vi "Init Condition.vi"(5 "Sequencing":refnum<class "MessageQ.lvclass">, 6 "Variables":refnum<class "Variables.lvclass">, 7 "VolatusAPI":refnum<class "VolatusAPI.lvclass">, 8 "error in (no error)":refnum<class "MultiErrors.lvclass">, 10 "Condition Config":refnum<class "Condition Config.lvclass">, 11 "OutOfRange Condition in":refnum<class "OutOfRange Condition.lvclass">) -> (0 "error out":refnum<class "MultiErrors.lvclass">, 3 "OutOfRange Condition out":refnum<class "OutOfRange Condition.lvclass">)   [LabVIEW 2020, in "VolatusSeq.lvlib" / "OutOfRange Condition.lvclass"]
uses:
  OutOfRange Condition.lvclass
  VolatusErrorUtilities/MultiErrors/MultiErrors.lvclass
  Volatus/VolatusAPI/VolatusAPI.lvclass
  VolatusSeqConfig/Condition Config/Condition Config.lvclass
  Volatus/MessageQ/MessageQ.lvclass
  VolatusSeqConfig/OutOfRange Condition Config/OutOfRange Condition Config.lvclass
  Volatus/VolatusAPI/VolatusAPI.lvclass/VolatusAPI.ctl
  OutOfRange Condition.lvclass/OutOfRange Condition.ctl
  lv-vecto/Vecto/ChannelService/Lookup Double Channel.vi
  Condition Value/Condition Value.lvclass
  Variables/Variables.lvclass
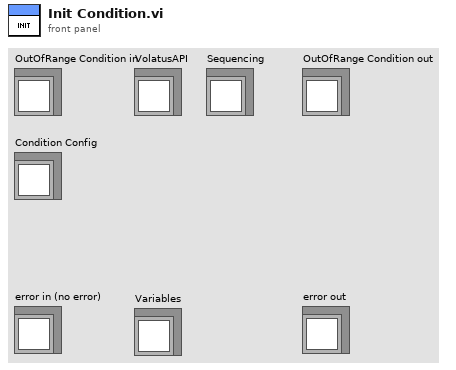
[diagram p1: front panel]
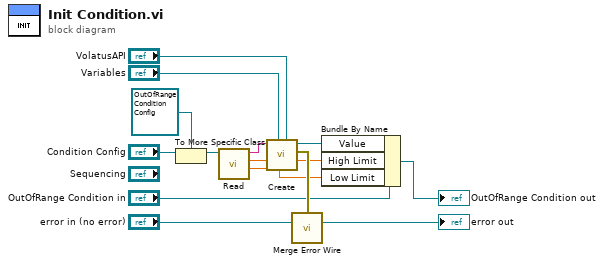
[diagram p0: block diagram]
diagram:
  n1 = To More Specific Class(target class=refnum<class "OutOfRange Condition Config.lvclass"> refnum ("VolatusSeqConfig.lvlib:OutOfRange Condition Config.lvclass"), reference="Condition Config") -> (specific class reference=w9:refnum<class "OutOfRange Condition Config.lvclass">)  [unwired: 1 in, 1 out]
  n2 = call "Read.vi"("OutOfRange Condition Config in"=w9) -> ("Low Limit"=w6:dbl, "High Limit"=w7:dbl, "Channel"=w3:string)  [unwired: 8 in]
  n3 = call "Create.vi"("VolatusAPI"="VolatusAPI", "Variables"="Variables", "Source Name"=w3) -> ("error out"=w14:errorcluster, "Condition Value out"=w4:refnum<class "Condition Value.lvclass">)  [unwired: 7 in]
  n4 = call "Merge Error Wire.vi"("error in (no error)"=w14, "MultiErrors in"="error in (no error)") -> ("MultiErrors out"=→"error out":refnum<class "MultiErrors.lvclass">)  [unwired: 13 in]
  n5 = Bundle By Name(cluster="OutOfRange Condition in", "Value"=w4, "High Limit"=w7, "Low Limit"=w6) -> (→"OutOfRange Condition out":refnum<class "OutOfRange Condition.lvclass">)
